vi "test motor sync fg.vi"() -> ()   [LabVIEW 2017]
uses:
  LV_Source/DataTypes/MotorSyncFGVAction--enum.ctl
panel:
  out "Status":cluster{"LA":bool, "TT":bool, "Osc":bool}
  out "MotorSync":bool
  in  "Motor":enum16{"LA", "TT", "Osc"}(ring)
  in  "update":bool
  in  "stop":bool
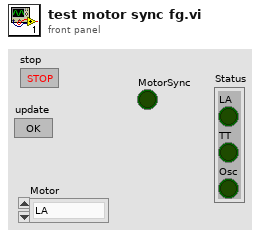
[diagram p1: front panel]
types:
  T1 = typedef "MotorSyncFGVAction--enum.ctl" = enum16{"Init", "Set", "Get"}
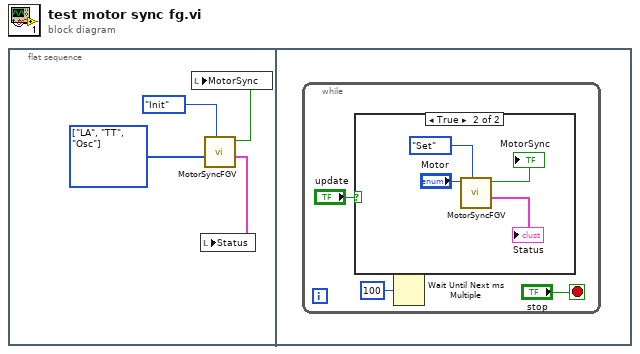
[diagram p0: block diagram]
diagram:
  n1 = flat-sequence {
    frame #0 {
      w3 = enum16{"LA", "TT", "Osc"}[] [enum."LA", enum."TT", enum."Osc"] items=["LA", "TT", "Osc"] ("MotorsToSync")
      n2 = call "MotorSyncFGV.vi"("Action_MotorSyncFGV"=MotorSyncFGVAction--enum."Init", "Initi MotorsToSync"=w3) -> ("Status"=w2:cluster{"LA":bool, "TT":bool, "Osc":bool}, "MotorSync"=w1:bool)  [unwired: 7 in, 1 out]
      n3 = local write "MotorSync"(w1) -> ()
      n4 = local write "Status"(w2) -> ()
    }
    frame #1 {
      n5 = while {
        stop <- "stop" stop-if-true
        n6 = case shown="True" "update" {
          frame False {
          }
          frame True {
            n7 = call "MotorSyncFGV.vi"("Action_MotorSyncFGV"=MotorSyncFGVAction--enum."Set", "Motor Select"="Motor") -> ("Status"=→"Status":cluster{"LA":bool, "TT":bool, "Osc":bool}, "MotorSync"=→"MotorSync":bool)  [unwired: 7 in, 1 out]
          }
        }
        n8 = Wait Until Next ms Multiple(millisecond multiple=u32 100) -> ()  [unwired: 1 out]
      }
    }
  }
